vi "Tag Metadata Write Tags Append.vi"(0 "Save Path":path, 7 "NameValues":string[][](array[string])) -> ()   [LabVIEW 2020]
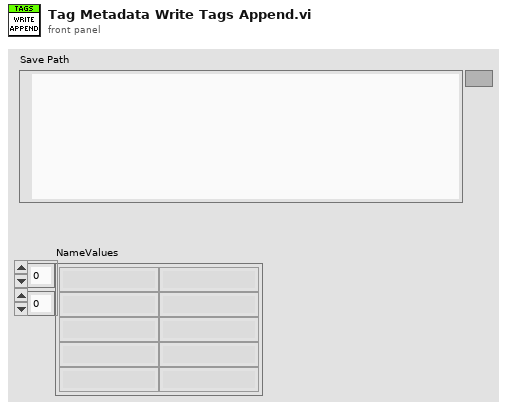
[diagram p1: front panel]
types:
  T1 = enum16{"open", "replace", "create", "open or create", "replace or create", "replace or create with confirmation"}
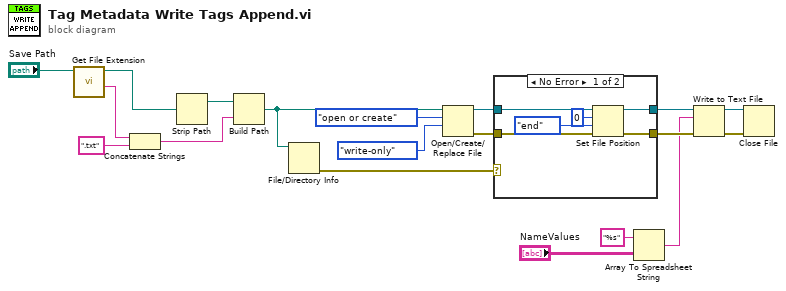
[diagram p0: block diagram]
diagram:
  n1 = call <vilib>:"Get File Extension.vi"("file"="Save Path") -> ("filename without extension"=w10:string, "dup file"=w9:path)  [unwired: 6 in, 3 out]
  n2 = Concatenate Strings(w10, ".txt" ("string")) -> (w11:string)
  n3 = Strip Path(path=w9) -> (stripped path=w8:path)  [unwired: 1 out]
  n4 = Build Path(base path=w8, name or relative path=w11) -> (appended path=w12:path)
  n5 = File/Directory Info(path=w12) -> (error out=w13:errorcluster)  [unwired: 1 in, 6 out]
  n6 = Open/Create/Replace File(file path (use dialog)=w12, operation (0:open)=T1."open or create", access (0:read/write)=enum16{"read/write", "read-only", "write-only"}."write-only") -> (refnum out=w14:refnum<file>, error out=w15:errorcluster)  [unwired: 3 in, 1 out]
  n7 = case shown="No Error" w13 {
    tunnel: w14 -> [w25 w27]
    tunnel: w15 -> [w22 w26]
    tunnel: [w21 w27] -> w16
    tunnel: [w20 w26] -> w17
    frame No Error {
      n8 = Set File Position(offset (in bytes) (0)=i64 0, refnum=w25, from (0:start)=enum16{"start", "end", "current"}."end", error in=w22) -> (refnum out=w21:refnum<file>, error out=w20:errorcluster)
    }
    frame Error {
    }
  }
  n9 = Array To Spreadsheet String(array="NameValues", 3:"%s" ("format string")) -> (spreadsheet string=w2:string)  [unwired: 1 in]
  n10 = Write to Text File(file (use dialog)=w16, text=w2, error in=w17) -> (refnum out=w18:refnum<file>, error out=w19:errorcluster)  [unwired: 1 in, 1 out]
  n11 = Close File(refnum=w18, error in=w19) -> ()  [unwired: 2 out]
